vi "LR-Interpolate-index.vi"(7 "Value":dbl format="%#_13g", 8 "error in (no error)":errorcluster, 9 "Lower index":i32, 10 "Previous":dbl format="%#_13g", 11 "Current":dbl format="%#_13g") -> (0 "error out":errorcluster, 1 "Fractional index":dbl format="%#_13g")   [LabVIEW 2013, in "HardwareCharacterization.lvlib" / "HC-LaserResponse.lvclass"]
doc: "Use this template to build a VI to use as a subVI."
uses:
  HC-LaserResponse.lvclass
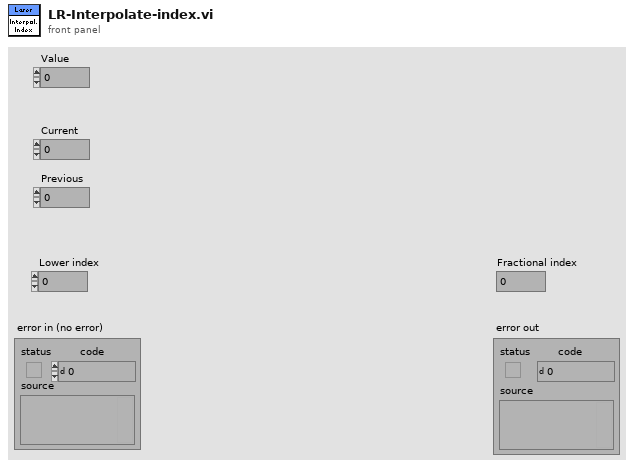
[diagram p1: front panel]
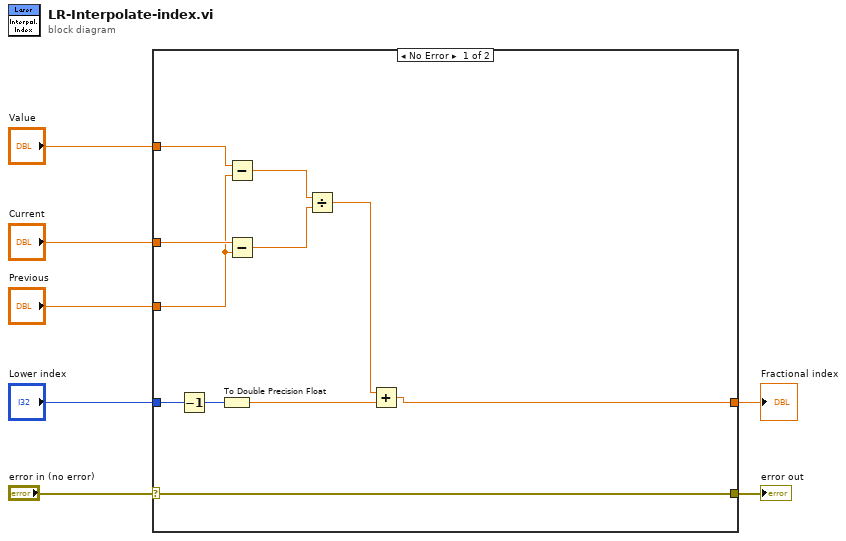
[diagram p0: block diagram]
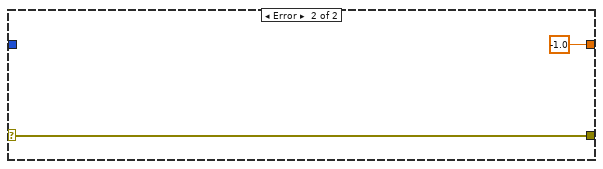
[diagram p2: hidden frame]
diagram:
  n1 = case shown="No Error" "error in (no error)" {
    selector: "error in (no error)" -> [w17 w20]
    tunnel: [w17 w20] -> w6
    tunnel: "Lower index" -> [w18 _]
    tunnel: "Previous" -> [w14 _]
    tunnel: "Current" -> [w15 _]
    tunnel: "Value" -> [w16 _]
    tunnel: [w9 -1.0] -> w1
    frame No Error {
      n2 = Decrement(x=w18) -> (x-1=w8:i32)
      n3 = To Double Precision Float(number=w8) -> (double precision float=w11:dbl)
      n4 = Subtract(x=w16, y=w14) -> (x-y=w13:dbl)
      n5 = Subtract(x=w15, y=w14) -> (x-y=w12:dbl)
      n6 = Divide(x=w13, y=w12) -> (x/y=w10:dbl)
      n7 = Add(x=w10, y=w11) -> (x+y=w9:dbl)
    }
    frame Error {
    }
  }
  "error out" <- w6
  "Fractional index" <- w1
